vi "ClockWiseReverse.vi"(8 "error in (no error)":errorcluster, 9 "index (row)":u16, 11 "Programming Logic in":refnum<class "Programming Logic.lvclass">) -> (0 "error out":errorcluster, 3 "Programming Logic out":refnum<class "Programming Logic.lvclass">, 10 "Direction":string)   [LabVIEW 2014, in "Files Library.lvlib"]
uses:
  Files Library.lvlib
  Logic/Programming Logic.lvclass
panel:
  in  "array":string[][](array[string])
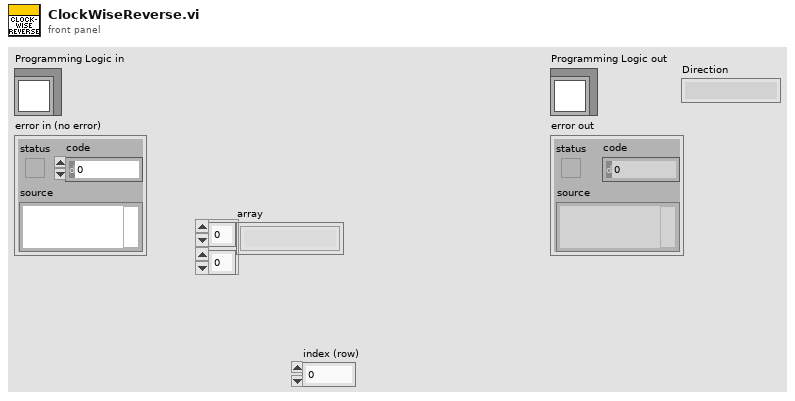
[diagram p1: front panel]
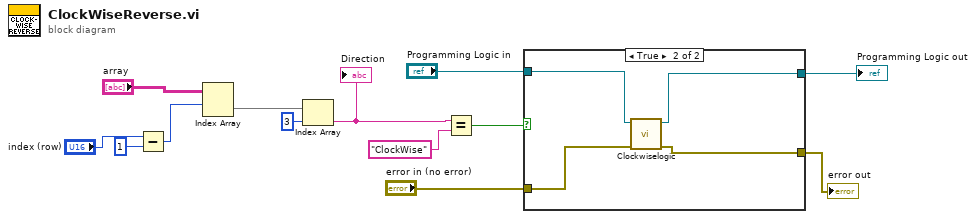
[diagram p0: block diagram]
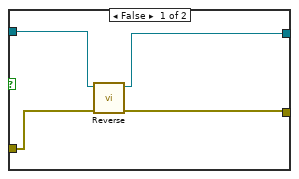
[diagram p2: hidden frame]
diagram:
  n1 = Subtract(x="index (row)", y=u16 1) -> (x-y=w1:u16)
  n2 = Index Array(array="array", index (row)=w1) -> (element=w11:string[])  [unwired: 1 in]
  n3 = Index Array(array=w11, index=3) -> (element=w8:string)
  "Direction" <- w8
  n4 = Equal?(x=w8, y="ClockWise") -> (x = y?=w10:bool)
  n5 = case shown="True" w10 {
    tunnel: [w16 w21] -> w7
    tunnel: "Programming Logic in" -> [w17 w20]
    tunnel: "error in (no error)" -> [w14 w19]
    tunnel: [w15 w18] -> w4
    frame False {
      n6 = call-dynamic "Reverse.vi"("error in (no error)"=w14, "Programming Logic in"=w17) -> ("error out"=w15:errorcluster, "Programming Logic out"=w16:refnum<class "Programming Logic.lvclass">)  [unwired: 8 in]
    }
    frame True {
      n7 = call-dynamic "Clockwiselogic.vi"("error in (no error)"=w19, "Programming Logic in"=w20) -> ("error out"=w18:errorcluster, "Programming Logic out"=w21:refnum<class "Programming Logic.lvclass">)  [unwired: 8 in]
    }
  }
  "Programming Logic out" <- w7
  "error out" <- w4
